vi "ELVIS III v1.0 RPC Register Heart Beat.vi"(8 "error in (no error)":errorcluster, 10 "Channel Names":string[](array[string]), 11 "Session":u32) -> (0 "error out":errorcluster)   [LabVIEW 2021]
uses:
  <vilib>/myRIO/Common/Instrument Driver Framework/ELVIS III v1.0/Resource Manager/typedefs/ELVIS III v1.0 RIO Session Map Action.ctl
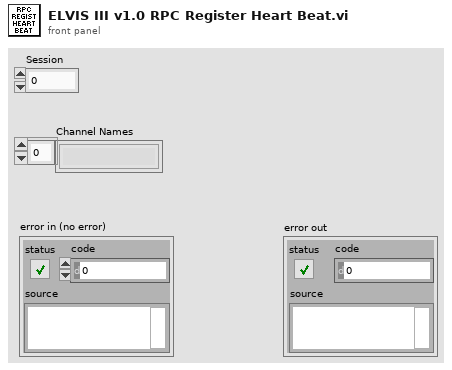
[diagram p1: front panel]
types:
  T1 = typedef "ELVIS III v1.0 RIO Session Map Action.ctl" = enum16{"Add Session", "Remove Session", "Get Active Sessions", "Get Owning Sessions"}
  T2 = enum32{"Bad", "Idle", "Run top level", "Running"}
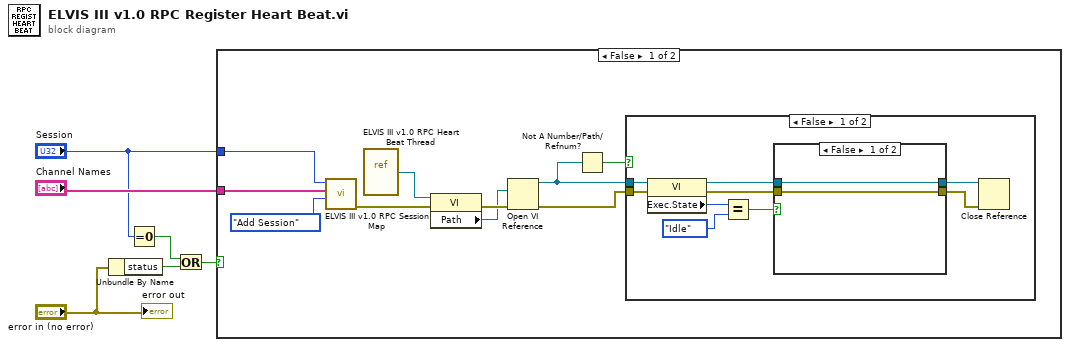
[diagram p0: block diagram]
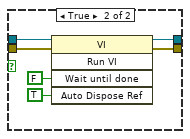
[diagram p2: hidden frame]
diagram:
  n1 = Unbundle By Name("error in (no error)") -> ("status"=w3:bool)
  n2 = Equal To 0?(x="Session") -> (x = 0?=w2:bool)
  n3 = Or(x=w2, y=w3) -> (x .or. y?=w1:bool)
  n4 = case shown="False" w1 {
    tunnel: "Session" -> [w16 _]
    tunnel: "Channel Names" -> [w8 _]
    frame False {
      n5 = call <vilib>:"ELVIS III v1.0 RPC Session Map.vi"("Action"=ELVIS_III_v1.0_RIO_Session_Map_Action."Add Session" ("Session Map Action"), "Channel Names"=w8, "Session"=w16) -> ("error out"=w12:errorcluster)  [unwired: 7 in, 1 out]
      n6 = vi-ref <vilib>:"ELVIS III v1.0 RPC Heart Beat Thread.vi"() -> (w13:refnum<vi>)
      n7 = property class="VI"(reference=w13, error in=w12) -> (error out=w15:errorcluster, "Path"=w14:path)  [unwired: 1 out]
      n8 = Open VI Reference(vi path=w14, error in (no error)=w15) -> (vi reference=w10:refnum<vi>, error out=w9:errorcluster)  [unwired: 4 in]
      n9 = Not A Number/Path/Refnum?(number/path/refnum=w10) -> (NaN/Path/Refnum?=w11:bool)
      n10 = case shown="False" w11 {
        tunnel: w10 -> [w25 _]
        tunnel: w9 -> [w17 _]
        frame False {
          n11 = property class="VI"(reference=w25, error in=w17) -> (reference out=w22:refnum<vi>, error out=w19:errorcluster, "Exec.State"=w23:T2)
          n12 = Equal?(x=w23, y=T2."Idle" ("Execution:State")) -> (x = y?=w21:bool)
          n13 = case shown="False" w21 {
            tunnel: w22 -> [w27 w33]
            tunnel: [w27 w30] -> w20
            tunnel: w19 -> [w26 w29]
            tunnel: [w26 w28] -> w18
            frame False {
            }
            frame True {
              n14 = invoke class="VI" method="Run VI"(reference=w33, error in=w29, "Wait until done"=FALSE ("Wait Until Done"), "Auto Dispose Ref"=TRUE ("Auto Dispose Reference")) -> (reference out=w30:refnum<vi>, error out=w28:errorcluster)  [unwired: 1 in, 3 out]
            }
          }
          n15 = Close Reference(reference=w20, error in (no error)=w18) -> ()  [unwired: 1 out]
        }
        frame True {
        }
      }
    }
    frame True {
      # "Session is invalid i.e. call from rpc server\nor error happens"
    }
  }
  "error out" <- "error in (no error)"
